vi "Create Arbitrary Waveform.vi"(6 "Timeout (10000)":i32=10000, 8 "error in (no error)":errorcluster, 9 "Arbitrary Waveform Data":dbl[](array[numeric]), 10 "Arbitrary Waveform Name (\"ARB1\")":string="ARB1", 11 "VISA resource name":refnum<visa-resource-name>) -> (0 "error out":errorcluster, 3 "VISA resource name out":refnum<visa-resource-name>)   [LabVIEW 2017, in "Agilent 33XXX Series.lvlib"]
doc: "Creates and saves an arbitrary (user-defined) waveform in non-volatile memory. \n\n<B>Note:</B>\n \n(1) Data is scaled and normalized so that the waveform will be centered around y=0. Models 33120A and 33250A have 12-bit digitizers and will be scaled from -2047 to +2047. Model 33210A and 33220A has a 14-bit digitizer and will be scaled from -8191 to + 8191.\n\n(2) Call Configure Arbitrary Waveform VI to set the arbitrary waveform as the active function.\n\n(3) Creates an arbitrary waveform in non-volatile memory and because of this, the waveform will remain stored on the instrument until deleted. If any sensitive information is contained in the arbitrary waveform, it is recommended that the waveform be deleted when finished"
uses:
  Agilent 33XXX Series.lvlib
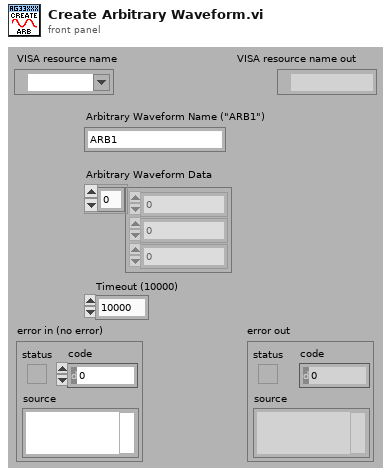
[diagram p1: front panel]
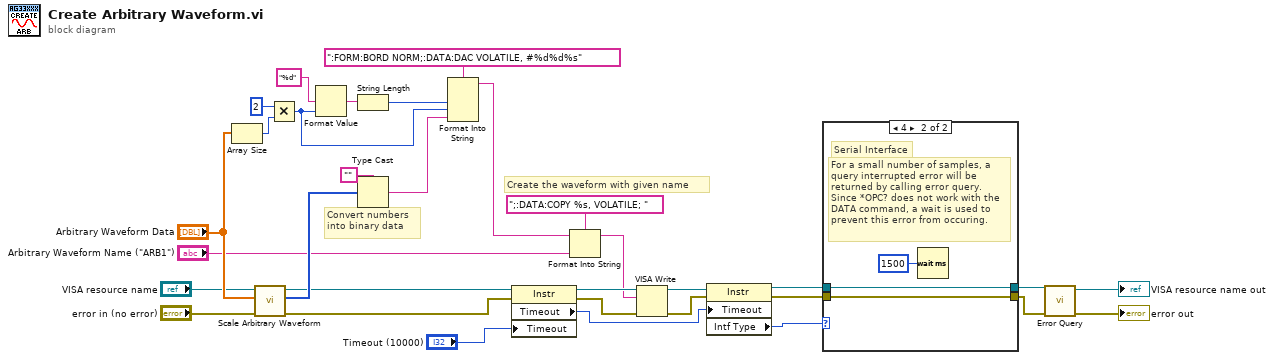
[diagram p0: block diagram]
diagram:
  # "Convert numbers\ninto binary data"
  # "Create the waveform with given name"
  n1 = Array Size(array="Arbitrary Waveform Data") -> (size(s)=w31:i32)
  n2 = call "Scale Arbitrary Waveform.vi"("error in (no error)"="error in (no error)", "Arbitrary Waveform Data"="Arbitrary Waveform Data", "VISA resource name"="VISA resource name") -> ("error out"=w24:errorcluster, "Scaled Arbitrary Waveform Data"=w26:i16[], "VISA resource name out"=w25:refnum<visa-resource-name>)  [unwired: 6 in]
  n3 = Multiply(x=2, y=w31) -> (x*y=w15:i32)
  n4 = Format Value(format string="%d", value (0)=w15) -> (output string=w28:string)  [unwired: 1 in]
  n5 = String Length(string=w28) -> (length=w16:i32)
  n6 = Type Cast(type="" ("Empty String Constant"), x=w26) -> (*(type *) &x=w14:string)
  n7 = Format Into String(format string=":FORM:BORD NORM;:DATA:DAC VOLATILE, #%d%d%s" ("string"), w16, w15, w14) -> (resulting string=w12:string)  [unwired: 2 in, 1 out]
  n8 = property on="Property Node" class="Instr"(reference=w25, error in=w24, "Timeout"="Timeout (10000)") -> (reference out=w22:refnum<visa-resource-name>, error out=w23:errorcluster, "Timeout"=w19:u32)
  n9 = Format Into String(format string=";:DATA:COPY %s, VOLATILE; ", initial string=w12, "Arbitrary Waveform Name (\"ARB1\")") -> (resulting string=w10:string)  [unwired: 1 in, 1 out]
  n10 = VISA Write(VISA resource name=w22, write buffer=w10, error in (no error)=w23) -> (VISA resource name out=w21:refnum<visa-resource-name>, error out=w20:errorcluster)  [unwired: 1 out]
  n11 = property on="Property Node" class="Instr"(reference=w21, error in=w20, "Timeout"=w19) -> (reference out=w9:refnum<visa-resource-name>, error out=w7:errorcluster, "Intf Type"=w5:u16)
  n12 = case shown="4" w5 {
    tunnel: w9 -> [w34 w37]
    tunnel: [w34 w37] -> w8
    tunnel: w7 -> [w33 w36]
    tunnel: [w33 w36] -> w6
    frame 0, Default {
    }
    frame 4 {
      # "For a small number of samples, a query interrupted error will be returned by calling error query.  Since *OPC? does not work with the DATA command, a wait is used to prevent this error from occuring."
      # "Serial Interface"
      n13 = Wait (ms)(milliseconds to wait=u32 1500) -> ()  [unwired: 1 out]
    }
  }
  n14 = call "Error Query.vi"("error in (no error)"=w6, "VISA resource name"=w8) -> ("error out"=→"error out":errorcluster, "VISA resource name out"=→"VISA resource name out":refnum<visa-resource-name>)  [unwired: 6 in, 2 out]
